vi "readTestDescription.vi"(8 "error in (no error)":errorcluster, 11 "Prueba04 in":refnum<class "Prueba04.lvclass">) -> (0 "error out":errorcluster, 2 "Test Description":string, 3 "Prueba04 out":refnum<class "Prueba04.lvclass">)   [LabVIEW 2019, in "Prueba04.lvclass"]
uses:
  Prueba04.lvclass
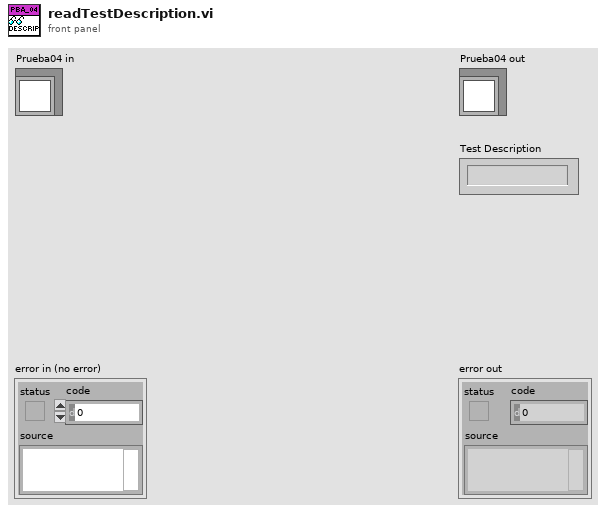
[diagram p1: front panel]
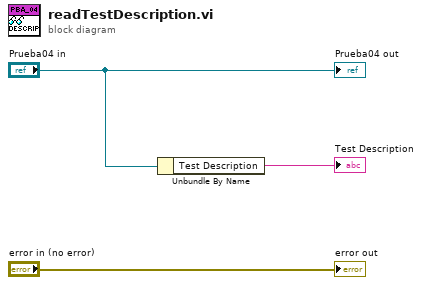
[diagram p0: block diagram]
diagram:
  n1 = Unbundle By Name("Prueba04 in") -> ("Test Description"=→"Test Description":string)
  "error out" <- "error in (no error)"
  "Prueba04 out" <- "Prueba04 in"
